vi "Get Control Indicator ref.vi"(8 "error in":errorcluster, 11 "panel refnum":refnum<vi>) -> (0 "error out":errorcluster, 2 "Indicators[]":refnum<vi>[](array[refnum]), 3 "Controls[]":refnum<vi>[](array[refnum]))   [LabVIEW 2020, in "Measurement Client Wrapper.lvclass"]
uses:
  Measurement Client Wrapper.lvclass
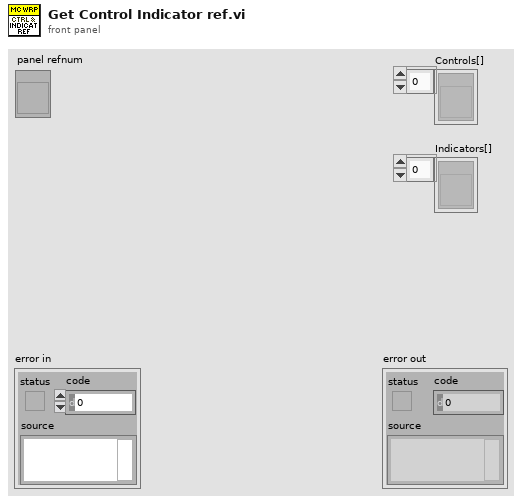
[diagram p1: front panel]
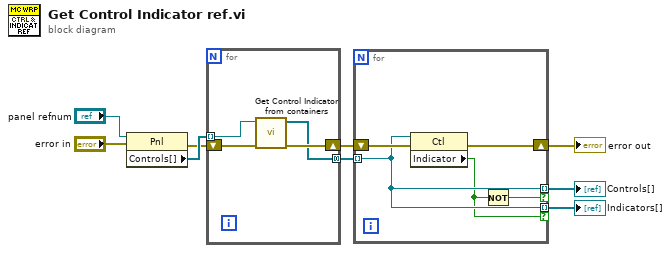
[diagram p0: block diagram]
diagram:
  n1 = property class="Pnl"(reference="panel refnum", error in="error in") -> (error out=w6:errorcluster, "Controls[]"=w9:refnum<vi>[])  [unwired: 1 out]
  n2 = for {
    tunnel: w9 -> [w12] mode=indexing
    tunnel: [w10] -> w5 mode=concatenating
    shift-right: [w11] -> w4
    shift-left: w6 -> [w13]
    n3 = call "Get Control Indicator from containers.vi"("error in"=w13, "Control ref"=w12) -> ("error out"=w11:errorcluster, "Controls[]"=w10:refnum<vi>[])  [unwired: 8 in]
  }
  n4 = for {
    tunnel: w5 -> [w16] mode=indexing
    shift-right: [w17] -> w1
    shift-left: w4 -> [w18]
    tunnel: [w16] -> w3 mode=indexing if=w14
    tunnel: [w16] -> w2 mode=indexing if=w15
    n5 = property class="Ctl"(reference=w16, error in=w18) -> (error out=w17:errorcluster, "Indicator"=w15:bool)  [unwired: 1 out]
    n6 = Not(x=w15) -> (.not. x?=w14:bool)
  }
  "error out" <- w1
  "Controls[]" <- w3
  "Indicators[]" <- w2
